vi "String Text Format by Tag.vi"(9 "String in":string, 11 "String Ref in":refnum<vi>) -> (3 "String Ref out":refnum<vi>)   [LabVIEW 2014]
doc: "<b>VI Type:</b> Standard VI \n<b>VI Description:</b> This VI loads a string control or indicator with a fomatted text string. The formatting options, Bold, Italics, Underline, & Strikethrough, are controlled by the use of inline tags as listed below. Wire the String Ref In input with the reference to the string control you wish to format. Wire the Text input with the text with format tags you want to use. The VI will load the control as it formats the contents. Loading the control directly could cause odd behavior with appearance.\n\nText Tag for Formatting\n\n<B> Bold </B>\n<I> Italic </I>\n<U> Underline </U>\n<S> Strikeout </S>"
uses:
  <vilib>/Utility/miscctls.llb/LVSelectionTypeDef.ctl
panel:
  out "Text":T1(array[cluster])
  in  "Style":T2(ring)
  # "Text Tag\n\n<B> Bold </B>\n<I> Italic </I>\n<U> Underline </U>\n<S> Strikeout </S>"
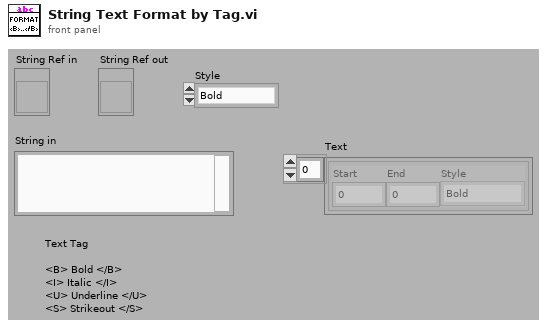
[diagram p1: front panel]
types:
  T1 = cluster{"Start":i32, "End":i32, "Style":enum16{"Bold", "Italic", "Underline", "Strikeout"}}[]
  T2 = enum16{"Bold", "Italic", "Underline", "Strikeout"}
  T3 = typedef "LVSelectionTypeDef.ctl" = cluster{"Selection Start":u32, "Selection End":u32}
  T4 = cluster{"Start":i32, "End":i32, "Style":enum16{"Bold", "Italic", "Underline", "Strikeout"}}
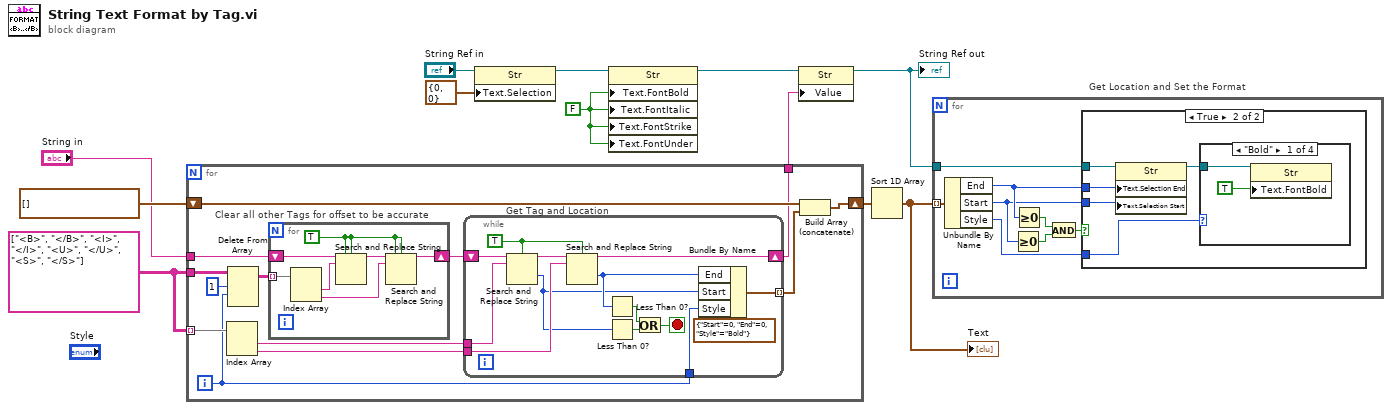
[diagram p0: block diagram]
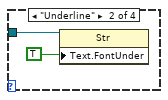
[diagram p3: hidden frame]
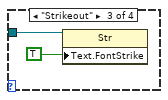
[diagram p4: hidden frame]
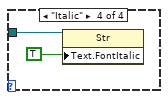
[diagram p5: hidden frame]
diagram:
  w12 = FALSE
  w5 = string[][] [["<B>", "</B>"], ["<I>", "</I>"], ["<U>", "</U>"], ["<S>", "</S>"]]
  # "Get Location and Set the Format"
  n1 = for {
    tunnel: w5 -> [w21] mode=indexing
    shift-right: [w23] -> w10
    shift-left: T1 [] ("Array") -> [w22]
    tunnel: w5 -> [w20]
    tunnel: "String in" -> [w17]
    tunnel: [w13] -> w4
    i -> [w15]
    # "Get Tag and Location"
    # "Clear all other Tags for offset to be accurate"
    n2 = Index Array(array=w21) -> (element #1=w25:string, element #2=w24:string)  [unwired: 2 in]
    n3 = Delete From Array(array=w20, length=1, index (row)=w15) -> (array with subset deleted=w18:string[][])  [unwired: 1 in, 1 out]
    n4 = for {
      shift-right: [w30] -> w19
      shift-left: w17 -> [w31]
      tunnel: w18 -> [w29] mode=indexing
      w26 = TRUE ("ignore case? (F)")
      n5 = Index Array(array=w29) -> (element #1=w28:string, element #2=w27:string)  [unwired: 2 in]
      n6 = Search and Replace String(replace all?=w26, case sensitive?=w26, input string=w31, search string=w28) -> (result string=w32:string)  [unwired: 1 in, 6 out]
      n7 = Search and Replace String(replace all?=w26, case sensitive?=w26, input string=w32, search string=w27) -> (result string=w30:string)  [unwired: 1 in, 6 out]
    }
    n8 = while {
      shift-right: [w44] -> w13
      shift-left: w19 -> [w46]
      tunnel: w25 -> [w42]
      tunnel: w24 -> [w41]
      tunnel: w15 -> [w36]
      tunnel: [w33] -> w14 mode=indexing
      stop <- w38 stop-if-true
      w43 = TRUE ("ignore case? (F)")
      n9 = Search and Replace String(case sensitive?=w43, input string=w46, search string=w42) -> (result string=w45:string, offset past replacement=w34:i32)  [unwired: 1 in, 6 out]
      n10 = Search and Replace String(case sensitive?=w43, input string=w45, search string=w41) -> (result string=w44:string, offset past replacement=w35:i32)  [unwired: 1 in, 6 out]
      n11 = Less Than 0?(x=w35) -> (x < 0?=w40:bool)
      n12 = Less Than 0?(x=w34) -> (x < 0?=w39:bool)
      n13 = Or(x=w40, y=w39) -> (x .or. y?=w38:bool)
      n14 = Bundle By Name(cluster=T4 {"Start"=0, "End"=0, "Style"=enum."Bold"} ("Cluster"), "End"=w35, "Start"=w34, "Style"=w36) -> (w33:T4)
    }
    n15 = Build Array (concatenate)(w22, w14) -> (w23:T1)
  }
  n16 = property class="Str"(reference="String Ref in", "Text.Selection"=T3 {"Selection Start"=0, "Selection End"=0}) -> (reference out=w6:refnum<vi>)  [unwired: 1 in, 1 out]
  n17 = property class="Str"(reference=w6, "Text.FontBold"=w12, "Text.FontItalic"=w12, "Text.FontStrike"=w12, "Text.FontUnder"=w12) -> (reference out=w3:refnum<vi>)  [unwired: 1 in, 1 out]
  n18 = property class="Str"(reference=w3, "Value"=w4) -> (reference out=w2:refnum<vi>)  [unwired: 1 in, 1 out]
  "String Ref out" <- w2
  n19 = Sort 1D Array(array=w10) -> (sorted array=w9:T1)
  "Text" <- w9
  n20 = for {
    tunnel: w9 -> [w54] mode=indexing
    tunnel: w2 -> [w48]
    n21 = Unbundle By Name(w54) -> ("End"=w50:i32, "Start"=w49:i32, "Style"=w47:T2)
    n22 = Greater Or Equal To 0?(x=w49) -> (x >= 0?=w52:bool)
    n23 = Greater Or Equal To 0?(x=w50) -> (x >= 0?=w53:bool)
    n24 = And(x=w53, y=w52) -> (x .and. y?=w51:bool)
    n25 = case shown="True" w51 {
      tunnel: w48 -> [_ w59]
      tunnel: w50 -> [_ w58]
      tunnel: w49 -> [_ w57]
      tunnel: w47 -> [_ w55]
      frame False {
      }
      frame True {
        n26 = property class="Str"(reference=w59, "Text.Selection End"=w58, "Text.Selection Start"=w57) -> (reference out=w56:refnum<vi>)  [unwired: 1 in, 1 out]
        n27 = case shown="\"Bold\"" w55 {
          tunnel: w56 -> [w61 w63 w65 w67]
          frame "Bold" {
            n28 = property class="Str"(reference=w61, "Text.FontBold"=TRUE ("Text.Font:Bold")) -> ()  [unwired: 1 in, 2 out]
          }
          frame "Underline" {
            n29 = property class="Str"(reference=w63, "Text.FontUnder"=TRUE ("Text.Font:Bold")) -> ()  [unwired: 1 in, 2 out]
          }
          frame "Strikeout" {
            n30 = property class="Str"(reference=w65, "Text.FontStrike"=TRUE ("Text.Font:Bold")) -> ()  [unwired: 1 in, 2 out]
          }
          frame "Italic" {
            n31 = property class="Str"(reference=w67, "Text.FontItalic"=TRUE ("Text.Font:Bold")) -> ()  [unwired: 1 in, 2 out]
          }
        }
      }
    }
  }
